vi "iHR550 Connect.vi"(0 "Force\nInitialization":bool, 2 "Grating Selector":refnum<vi>, 3 "Mono ID":string(combo)="Mono4") -> (5 "Emulating":bool, 6 "Initialized":bool=TRUE, 7 "iHR550 Error Out":errorcluster, 8 "Current Description":string="1", 9 "Current Grating":dbl=1200.0, 10 "iHR550 RefNum":refnum<k7> caption="Mono RefNum out")   [LabVIEW 2010]
panel:
  out "Status":string="Initialized"
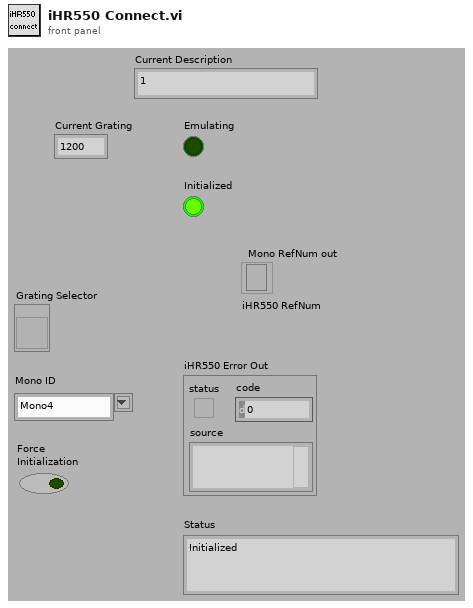
[diagram p1: front panel]
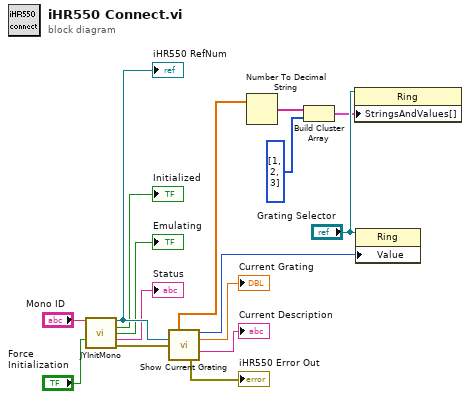
[diagram p0: block diagram]
diagram:
  n1 = call "JYInitMono.vi"("Unique ID"="Mono ID", "Force Init"="Force\nInitialization") -> ("Mono RefNum out"=w14:refnum<k7>, "Initialized"=→"Initialized":bool, "Emulating"=→"Emulating":bool, "Status"=→"Status":string, "error out"=w15:errorcluster)  [unwired: 9 in]
  "iHR550 RefNum" <- w14
  n2 = call "Show Current Grating.vi"("Refnum in"=w14, "error in (no error)"=w15) -> ("Gratings"=w13:dbl[], "Grating Index"=w4:i32, "Current Grating"=→"Current Grating":dbl, "Current Description"=→"Current Description":string, "error out"=→"iHR550 Error Out":errorcluster)  [unwired: 5 in, 4 out]
  n3 = Number To Decimal String(number=w13) -> (decimal integer string=w2:string[])  [unwired: 1 in]
  n4 = Build Cluster Array(w2, i32[] [1, 2, 3] ("Element")) -> (w1:cluster{"Numeric":string, i32}[])
  n5 = property on="Eigenschaftsknoten" class="Ring"(reference="Grating Selector", "StringsAndValues[]"=w1) -> ()  [unwired: 1 in, 2 out]
  n6 = property on="Eigenschaftsknoten" class="Ring"(reference="Grating Selector", "Value"=w4) -> ()  [unwired: 1 in, 2 out]
